vi "Read AcroFields.vi"() -> ()   [LabVIEW 2019, in "Exaprom PDF.lvlib"]
uses:
  Controls/AcroField.ctl
  C:/work/niobrara_lv/labview pdf writer fixing/DLL/itextsharp.dll
  DLL/itextsharp.dll
  Exaprom PDF.lvlib
panel:
  in  "error in (no error)":errorcluster
  out "Key and Value [ ]":T1[](array[typedef])
  out "error out":errorcluster
  in  "path":path
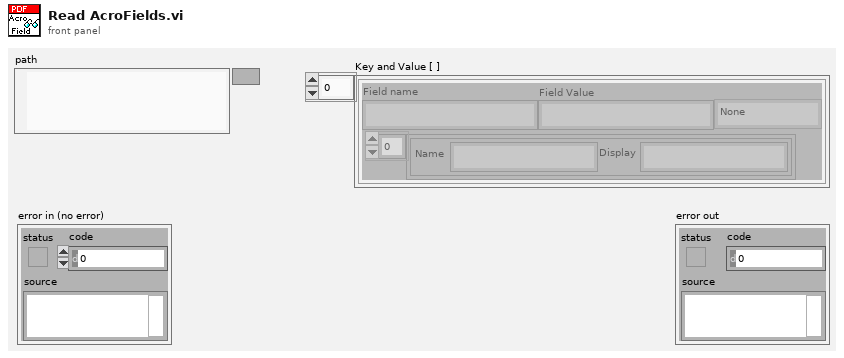
[diagram p1: front panel]
types:
  T1 = typedef "Exaprom PDF.lvlib/AcroField.ctl" = cluster{"Field name":string, "Field Value":string, "Type":enum16{"None", "Push Button", "CheckBox", "RadioButton", "Text", "List", "Combo", "Signature"}, "Name [ ]":cluster{"Name":string, "Display":string}[]}
  T2 = cluster{"ToString":string, "GetField":string, "GetFieldType":i32, "Value [ ]":cluster{"Value":string, "Display":string}[]}
  T3 = cluster{"ToString":string, "GetField":string, "GetFieldType":i32, "Value [ ]":cluster{"Value":string, "Display":string}[]}[]
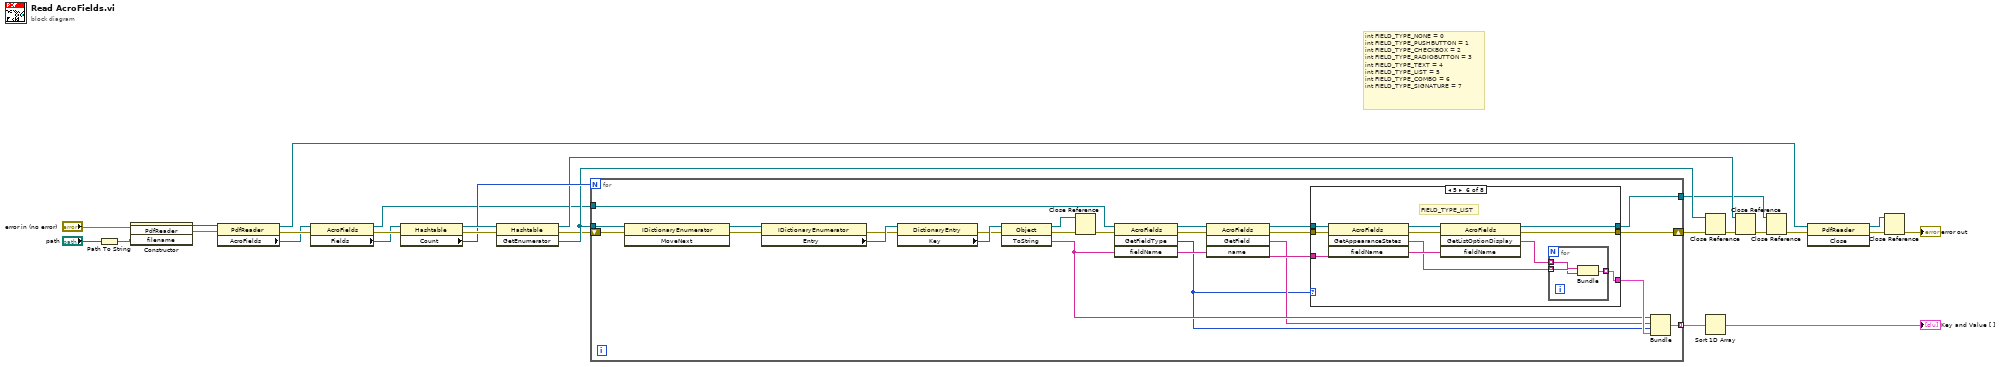
[diagram p0: block diagram]
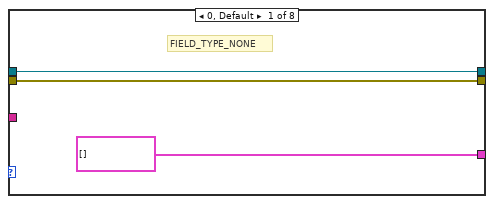
[diagram p2: hidden frame]
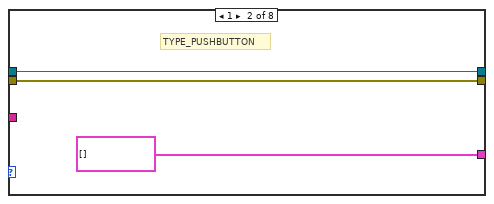
[diagram p3: hidden frame]
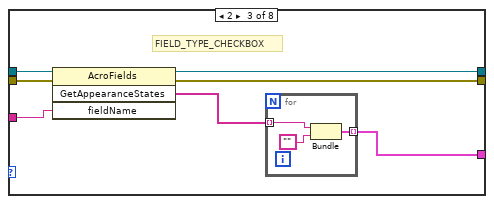
[diagram p4: hidden frame]
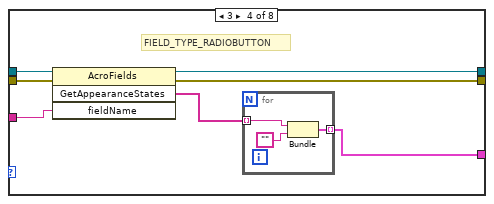
[diagram p5: hidden frame]
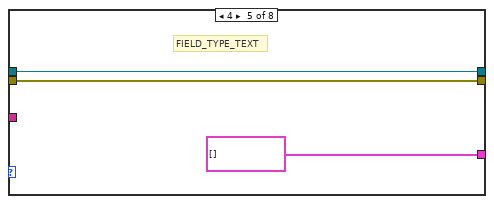
[diagram p6: hidden frame]
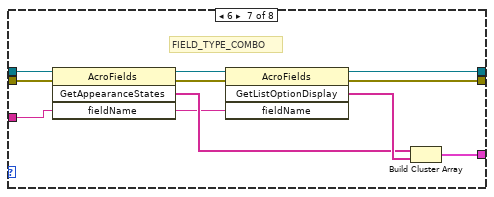
[diagram p7: hidden frame]
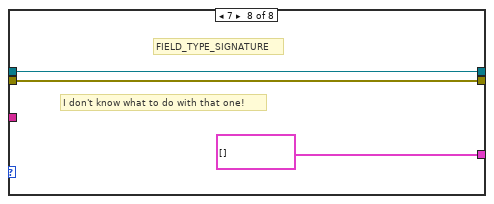
[diagram p8: hidden frame]
diagram:
  # "int FIELD_TYPE_NONE = 0\nint FIELD_TYPE_PUSHBUTTON = 1\nint FIELD_TYPE_CHECKBOX = 2\nint FIELD_TYPE_RADIOBUTTON = 3\nint FIELD_TYPE_TEXT = 4\nint FIELD_TYPE_LIST = 5\nint FIELD_TYPE_COMBO = 6\nint FIELD_TYPE_SIGNATURE = 7"
  n1 = Path To String(path="path") -> (string=w27:string)
  n2 = constructor class="PdfReader"(error in="error in (no error)", "filename"=w27) -> (reference out=w26:refnum<k24>, error out=w24:errorcluster)  [unwired: 2 in, 2 out]
  n3 = property class="PdfReader"(reference=w26, error in=w24) -> (reference out=w11:refnum<k24>, error out=w25:errorcluster, "AcroFields"=w6:refnum<k24>)
  n4 = property class="AcroFields"(reference=w6, error in=w25) -> (reference out=w5:refnum<k24>, error out=w22:errorcluster, "Fields"=w7:refnum<k24>)
  n5 = property class="Hashtable"(reference=w7, error in=w22) -> (reference out=w20:refnum<k24>, error out=w21:errorcluster, "Count"=w19:i32)
  n6 = invoke class="Hashtable" method="GetEnumerator"(reference=w20, error in=w21) -> (reference out=w15:refnum<k24>, error out=w1:errorcluster, "GetEnumerator"=w17:refnum<k24>)  [unwired: 1 in]
  n7 = for {
    N: w19 -> [_]
    tunnel: w17 -> [w48]
    tunnel: [w45] -> w18 mode=indexing
    tunnel: w5 -> [w41]
    tunnel: [w33] -> w2
    shift-right: [w34] -> w4
    shift-left: w1 -> [w29]
    n8 = invoke class="IDictionaryEnumerator" method="MoveNext"(reference=w48, error in=w29) -> (reference out=w46:refnum<k24>, error out=w47:errorcluster)  [unwired: 1 in, 1 out]
    n9 = property class="IDictionaryEnumerator"(reference=w46, error in=w47) -> (error out=w49:errorcluster, "Entry"=w50:refnum<k24>)  [unwired: 1 out]
    n10 = property class="DictionaryEntry"(reference=w50, error in=w49) -> (error out=w28:errorcluster, "Key"=w44:refnum<k24>)  [unwired: 1 out]
    n11 = invoke class="Object" method="ToString"(reference=w44, error in=w28) -> (reference out=w43:refnum<k24>, error out=w40:errorcluster, "ToString"=w32:string)  [unwired: 1 in]
    n12 = Close Reference(reference=w43, error in (no error)=w40) -> (error out=w42:errorcluster)
    n13 = invoke class="AcroFields" method="GetFieldType"(reference=w41, error in=w42, "fieldName"=w32) -> (reference out=w35:refnum<k24>, error out=w38:errorcluster, "GetFieldType"=w30:i32)  [unwired: 1 in, 1 out]
    n14 = invoke class="AcroFields" method="GetField"(reference=w35, error in=w38, "name"=w32) -> (reference out=w36:refnum<k24>, error out=w37:errorcluster, "GetField"=w31:string)  [unwired: 1 in, 1 out]
    n15 = case shown="5" w30 {
      tunnel: [cluster{"Value":string, "Display":string}[] [] ("Value [ ]") cluster{"Value":string, "Display":string}[] [] ("Value [ ]") w58 w67 cluster{"Value":string, "Display":string}[] [] ("Value [ ]") w80 w100 cluster{"Value":string, "Display":string}[] [] ("Value [ ]")] -> w39
      tunnel: [w52 w55 w62 w72 w78 w84 w94 w104] -> w34
      tunnel: w37 -> [w52 w55 w63 w73 w78 w89 w102 w104]
      tunnel: w36 -> [w51 w54 w57 w71 w77 w88 w101 w103]
      tunnel: w32 -> [_ _ w61 w70 _ w85 w95 _]
      tunnel: [w51 w54 w60 w69 w77 w83 w93 w103] -> w33
      frame 0, Default {
        # "FIELD_TYPE_NONE"
      }
      frame 1 {
        # "TYPE_PUSHBUTTON"
      }
      frame 2 {
        # "FIELD_TYPE_CHECKBOX"
        n16 = invoke class="AcroFields" method="GetAppearanceStates"(reference=w57, error in=w63, "fieldName"=w61) -> (reference out=w60:refnum<k24>, error out=w62:errorcluster, "GetAppearanceStates"=w59:string[])  [unwired: 1 in, 1 out]
        n17 = for {
          tunnel: w59 -> [w66] mode=indexing
          tunnel: [w64] -> w58 mode=indexing
          n18 = Bundle(w66, "") -> (w64:cluster{string, string})  [unwired: 1 in]
        }
      }
      frame 3 {
        # "FIELD_TYPE_RADIOBUTTON"
        n19 = invoke class="AcroFields" method="GetAppearanceStates"(reference=w71, error in=w73, "fieldName"=w70) -> (reference out=w69:refnum<k24>, error out=w72:errorcluster, "GetAppearanceStates"=w68:string[])  [unwired: 1 in, 1 out]
        n20 = for {
          tunnel: w68 -> [w76] mode=indexing
          tunnel: [w74] -> w67 mode=indexing
          n21 = Bundle(w76, "") -> (w74:cluster{string, string})  [unwired: 1 in]
        }
      }
      frame 4 {
        # "FIELD_TYPE_TEXT"
      }
      frame 5 {
        # "FIELD_TYPE_LIST"
        n22 = invoke class="AcroFields" method="GetAppearanceStates"(reference=w88, error in=w89, "fieldName"=w85) -> (reference out=w87:refnum<k24>, error out=w86:errorcluster, "GetAppearanceStates"=w82:string[])  [unwired: 1 in, 1 out]
        n23 = invoke class="AcroFields" method="GetListOptionDisplay"(reference=w87, error in=w86, "fieldName"=w85) -> (reference out=w83:refnum<k24>, error out=w84:errorcluster, "GetListOptionDisplay"=w81:string[])  [unwired: 1 in, 1 out]
        n24 = for {
          tunnel: w82 -> [w92] mode=indexing
          tunnel: [w91] -> w80 mode=indexing
          tunnel: w81 -> [w90] mode=indexing
          n25 = Bundle(w92, w90) -> (w91:cluster{string, string})  [unwired: 1 in]
        }
      }
      frame 6 {
        # "FIELD_TYPE_COMBO"
        n26 = invoke class="AcroFields" method="GetAppearanceStates"(reference=w101, error in=w102, "fieldName"=w95) -> (reference out=w99:refnum<k24>, error out=w98:errorcluster, "GetAppearanceStates"=w96:string[])  [unwired: 1 in, 1 out]
        n27 = invoke class="AcroFields" method="GetListOptionDisplay"(reference=w99, error in=w98, "fieldName"=w95) -> (reference out=w93:refnum<k24>, error out=w94:errorcluster, "GetListOptionDisplay"=w97:string[])  [unwired: 1 in, 1 out]
        n28 = Build Cluster Array(w96, w97) -> (w100:cluster{string, string}[])
      }
      frame 7 {
        # "I don't know what to do with that one!"
        # "FIELD_TYPE_SIGNATURE"
      }
    }
    n29 = Bundle("ToString"=w32, "GetField"=w31, "GetFieldType"=w30, "Value [ ]"=w39) -> (w45:T2)  [unwired: 1 in]
  }
  n30 = Close Reference(reference=w17, error in (no error)=w4) -> (error out=w16:errorcluster)
  n31 = Sort 1D Array(array=w18) -> (sorted array=→"Key and Value [ ]":T3)
  n32 = Close Reference(reference=w15, error in (no error)=w16) -> (error out=w14:errorcluster)
  n33 = Close Reference(reference=w2, error in (no error)=w14) -> (error out=w13:errorcluster)
  n34 = invoke class="PdfReader" method="Close"(reference=w11, error in=w13) -> (reference out=w8:refnum<k24>, error out=w12:errorcluster)  [unwired: 1 in, 1 out]
  n35 = Close Reference(reference=w8, error in (no error)=w12) -> (error out=→"error out":errorcluster)
